vi "How to use in host.vi"(11 "Select Part":u16(ring) items=["P1.JPG", "P2.JPG", "P3.JPG", "P4.JPG", "P5.JPG", "P6.JPG", "P7.JPG", "P8.JPG", "P9.JPG", "P10.JPG", "P11.JPG", "P12.JPG"]) -> (0 "zoom":sgl, 1 "2D Picture":picture, 2 "output cluster":T1, 3 "Draw Area Size":T2={"Width"=554, "Height"=477})   [LabVIEW 2015]
uses:
  <vilib>/Utility/miscctls.llb/LVBoundsTypeDef.ctl
  <vilib>/Utility/miscctls.llb/LVPointTypeDef.ctl
  Galobal variable_TI.vi
panel:
  out "error out":errorcluster
  out "empty?":bool
  out "Out":T3(array[cluster])
  in  "stop":bool
  out "filenames":string[](array[string])
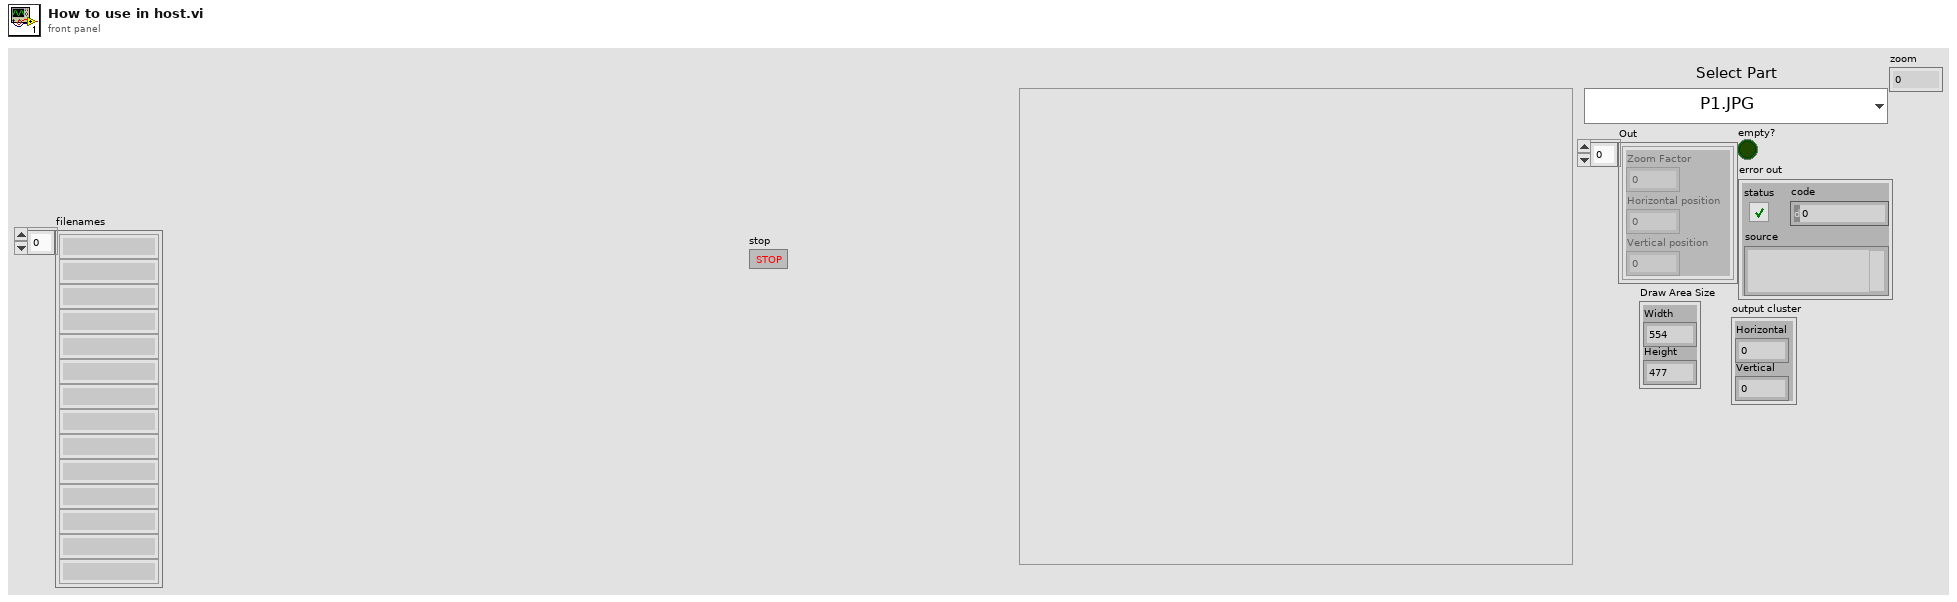
[diagram p1: front panel]
types:
  T1 = typedef "LVPointTypeDef.ctl" = cluster{"Horizontal":i16, "Vertical":i16}
  T2 = typedef "LVBoundsTypeDef.ctl" = cluster{"Width":u32, "Height":u32}
  T3 = cluster{"Zoom Factor":sgl, "Horizontal position":sgl, "Vertical position":sgl}[]
  T4 = typedef "imagedata.ctl" = cluster{"image type":i32, "image depth":i32, "image":u8[], "mask":u8[], "colors":u32[], "Rectangle":cluster{"left":i16, "top":i16, "right":i16, "bottom":i16}}
  T5 = cluster{"Zoom Factor":sgl, "Horizontal position":sgl, "Vertical position":sgl}
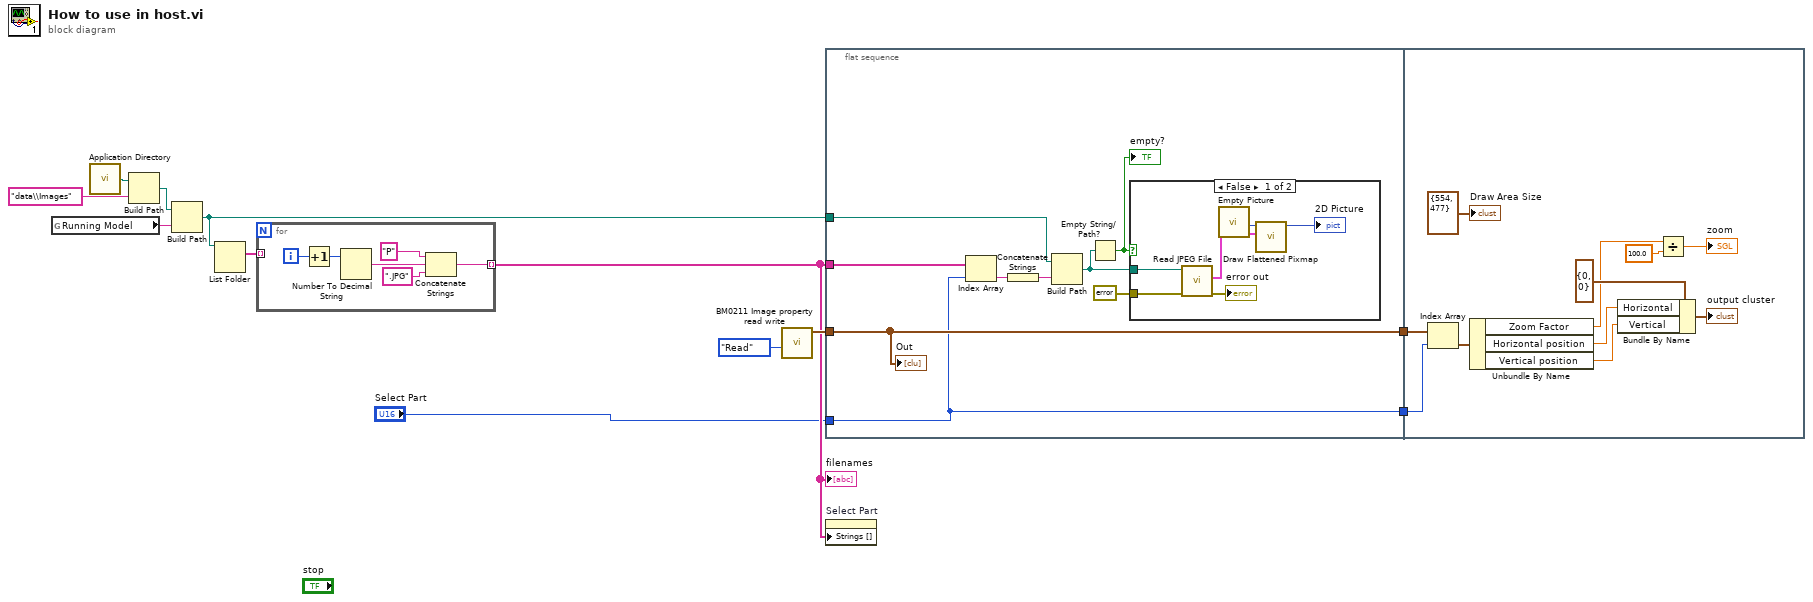
[diagram p0: block diagram]
diagram:
  n1 = global read "Galobal variable_TI.vi" "Running Model"() -> (w3:string)
  n2 = call <vilib>:"Application Directory.vi"() -> ("Application Directory"=w11:path)
  n3 = Build Path(base path=w11, name or relative path="data\\Images") -> (appended path=w4:path)
  n4 = Build Path(base path=w4, name or relative path=w3) -> (appended path=w2:path)
  n5 = List Folder(path=w2) -> (filenames=w6:string[])  [unwired: 3 in, 3 out]
  n6 = for {
    tunnel: [w14] -> w5 mode=indexing
    tunnel: w6 -> [_] mode=indexing
    i -> [w18]
    n7 = Increment(x=w18) -> (x+1=w13:i32)
    n8 = Number To Decimal String(number=w13) -> (decimal integer string=w16:string)  [unwired: 1 in]
    n9 = Concatenate Strings("P" ("string"), w16, ".JPG" ("string")) -> (w14:string)
  }
  "filenames" <- w5
  n10 = call "BM0211 Image property read write.vi"("Read write"=enum16{"write", "Read"}."Read") -> ("Out"=w9:T3)  [unwired: 9 in, 1 out]
  n11 = flat-sequence {
    tunnel: w5 -> [w26]
    tunnel: [w19] -> w8
    tunnel: [w24] -> w7
    tunnel: w9 -> [w24]
    tunnel: w2 -> [w20]
    tunnel: "Select Part" -> [w19]
    tunnel: w8 -> [w44]
    tunnel: w7 -> [w43]
    frame #0 {
      n12 = Index Array(array=w26, index=w19) -> (element=w25:string)
      n13 = Concatenate Strings(w25) -> (w27:string)
      n14 = Build Path(base path=w20, name or relative path=w27) -> (appended path=w23:path)
      n15 = Empty String/Path?(string/path=w23) -> (empty?=w22:bool)
      "empty?" <- w22
      n16 = case shown="False" w22 {
        tunnel: w23 -> [w30 _]
        tunnel: errorcluster {"status"=FALSE, "code"=0, "source"=""} ("error in (no error)") -> [w29 _]
        frame False {
          n17 = call <vilib>:"Read JPEG File.vi"("error in (no error)"=w29, "path to JPEG file"=w30) -> ("error out"=→"error out":errorcluster, "image data"=w32:T4)  [unwired: 7 in, 1 out]
          n18 = call "Empty Picture"() -> ("empty picture"=w33:picture)
          n19 = call <vilib>:"Draw Flattened Pixmap.vi"("image data"=w32, "picture"=w33) -> ("new picture"=→"2D Picture":picture)  [unwired: 7 in]
        }
        frame True {
        }
      }
      "Out" <- w24
    }
    frame #1 {
      n20 = Index Array(array=w43, index=w44) -> (element=w39:T5)
      n21 = Unbundle By Name(w39) -> ("Zoom Factor"=w37:sgl, "Horizontal position"=w41:sgl, "Vertical position"=w42:sgl)
      n22 = Bundle By Name(cluster=T1 {"Horizontal"=0, "Vertical"=0} ("Origin"), "Horizontal"=w41, "Vertical"=w42) -> (→"output cluster":T1)
      n23 = Divide(x=w37, y=sgl 100.0 ("x")) -> (x/y=→"zoom":sgl)
      "Draw Area Size" <- T2 {"Width"=554, "Height"=477} ("Draw Area Size")
    }
  }
  n24 = property on="Select Part" class="Ring (strict)"("Strings []"=w5) -> ()  [unwired: 2 in, 2 out]
